vi "Write AppOutput.vi"(8 "error in (no error)":errorcluster, 10 "AppOutput":variant, 11 "VisualizeAppBase_class in":refnum<class "VisualizeAppBase_class.lvclass">) -> (0 "error out":errorcluster, 3 "VisualizeAppBase_class out":refnum<class "VisualizeAppBase_class.lvclass">)   [LabVIEW 2014]
uses:
  VisualizeAppBase_class.lvclass
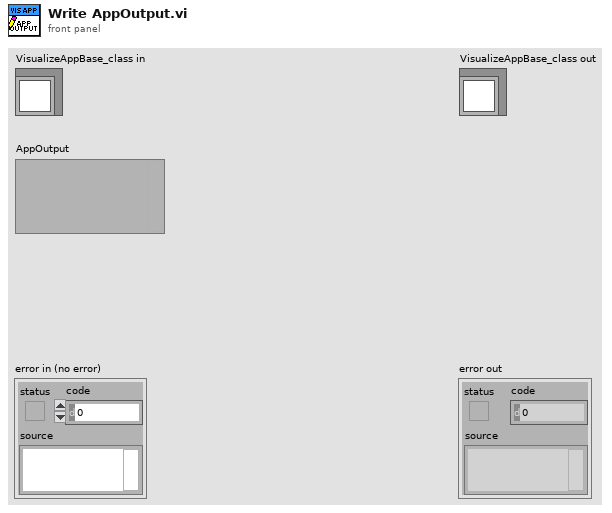
[diagram p1: front panel]
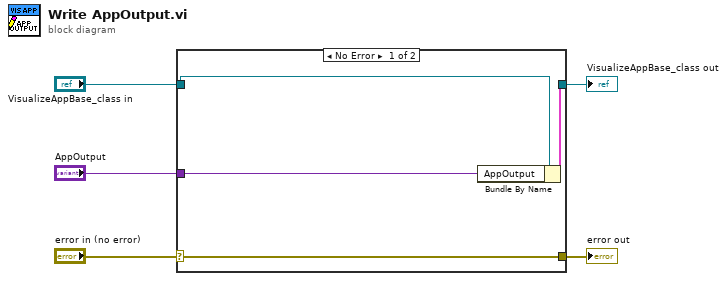
[diagram p0: block diagram]
diagram:
  n1 = case shown="No Error" "error in (no error)" {
    selector: "error in (no error)" -> [w9 w10]
    tunnel: [w9 w10] -> w4
    tunnel: [w7 w11] -> w2
    tunnel: "VisualizeAppBase_class in" -> [w8 w11]
    tunnel: "AppOutput" -> [w6 _]
    frame No Error {
      n2 = Bundle By Name(cluster=w8, "AppOutput"=w6) -> (w7:cluster{})
    }
    frame Error {
    }
  }
  "error out" <- w4
  "VisualizeAppBase_class out" <- w2
